vi "ParseArguments.vi"(8 "error in (no error)":errorcluster, 10 "DataReceived":refnum<class "DataReceived.lvclass">, 11 "Cli in":refnum<class "Cli.lvclass">) -> (0 "error out":errorcluster, 2 "Command":refnum<class "Command.lvclass">, 3 "Cli out":refnum<class "Cli.lvclass">)   [LabVIEW 2022 SP3, in "Cli.lvlib" / "Cli.lvclass"]
uses:
  Cli.lvclass
  Command/Command.lvclass
  Tcp/DataReceived/DataReceived.lvclass
  Cli.lvclass/Cli.ctl
  Tcp/DataReceived/DataReceived.lvclass/DataReceived.ctl
  Tcp/DataReceived/Read Data.vi
  ArgumentParser/Source/ArgumentParser/ArgumentParser.lvclass
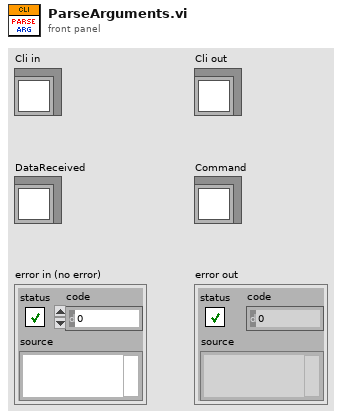
[diagram p1: front panel]
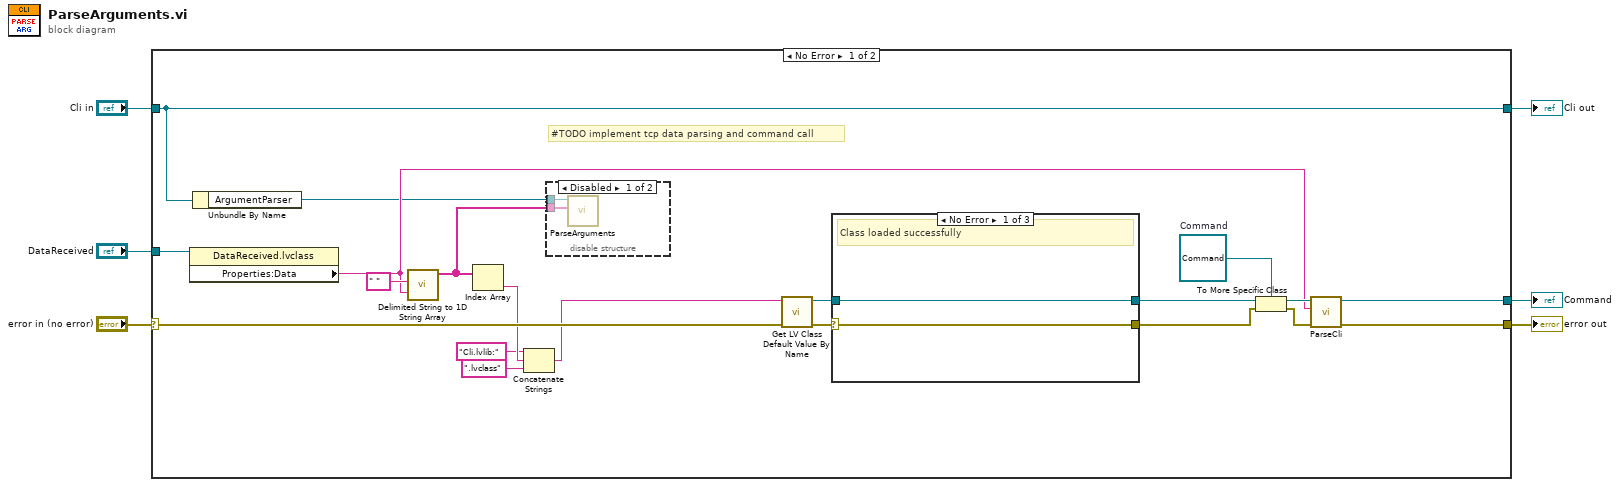
[diagram p0: block diagram]
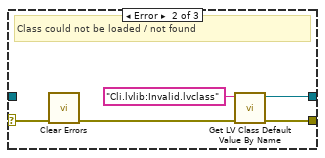
[diagram p3: hidden frame]
diagram:
  n1 = case shown="No Error" "error in (no error)" {
    selector: "error in (no error)" -> [w23 w39]
    tunnel: [w11 w39] -> w5
    tunnel: [w9 w38] -> w3
    tunnel: "Cli in" -> [w9 w38]
    tunnel: "DataReceived" -> [w26 _]
    tunnel: [w13 _] -> w1
    frame No Error {
      w24 = refnum<class "Command.lvclass"> refnum  # Command
      # "#TODO implement tcp data parsing and command call"
      n2 = property class="DataReceived.lvclass"(reference=w26) -> ("Properties:Data"=w10:string)  [unwired: 1 in, 2 out]
      n3 = Unbundle By Name(w9) -> ("ArgumentParser"=w8:refnum<class "ArgumentParser.lvclass">)
      n4 = call <vilib>:"Delimited String to 1D String Array.vi"("delimiter"=" ", "delimited string"=w10) -> ("string array"=w7:string[])  [unwired: 9 in]
      n5 = Index Array(array=w7) -> (element=w22:string)  [unwired: 1 in]
      n6 = Concatenate Strings("Cli.lvlib:" ("string"), w22, ".lvclass" ("string")) -> (w20:string)
      n7 = disable-structure shown="Disabled" {
        disable-tunnel: w8 -> [w28 _]
        disable-tunnel: w7 -> [w27 _]
        frame Disabled {
          n8 = call-dynamic "ParseArguments.vi"("CliArguments"=w27, "ArgumentParser in"=w28) -> ()  [unwired: 7 in, 3 out]
        }
        frame Enabled {
        }
      }
      n9 = call <vilib>:"Get LV Class Default Value By Name.vi"("error in (no error)"=w23, "class name"=w20) -> ("error out"=w18:errorcluster, "object"=w17:refnum<class>)  [unwired: 8 in]
      n10 = case shown="No Error" w18 {
        selector: w18 -> [w29 w35 w36]
        tunnel: w17 -> [w30 _ w37]
        tunnel: [w30 w32 w37] -> w16
        tunnel: [w29 w31 w36] -> w15
        frame No Error {
          # "Class loaded successfully"
        }
        frame Error {
          # "Class could not be loaded / not found"
          n11 = call <vilib>:"Clear Errors.vi"("error in (no error)"=w35) -> ("error out"=w34:errorcluster)  [unwired: 5 in, 1 out]
          n12 = call <vilib>:"Get LV Class Default Value By Name.vi"("error in (no error)"=w34, "class name"="Cli.lvlib:Invalid.lvclass") -> ("error out"=w31:errorcluster, "object"=w32:refnum<class>)  [unwired: 8 in]
        }
        frame Default {
          # "Error"
        }
      }
      n13 = To More Specific Class(target class=w24, reference=w16, error in=w15) -> (specific class reference=w14:refnum<class "Command.lvclass">, error out=w12:errorcluster)
      n14 = call-dynamic "ParseCli.vi"("error in (no error)"=w12, "Cli"=w10, "Command in"=w14) -> ("error out"=w11:errorcluster, "Command out"=w13:refnum<class "Command.lvclass">)  [unwired: 7 in]
    }
    frame Error {
    }
  }
  "error out" <- w5
  "Cli out" <- w3
  "Command" <- w1
